vi "OE1311&OE1351_Configure Demodulation.vi"(7 "OE1300_Configure Demodulator":T1={"Demodulator"=1, "Mode"=0, "Arbitrary Frequency"=1000.0, "Harmonic"=1, "Instrument Mode "=4, "Phase  (degree)"=0.0} {"Phase  (degree)" min=-180.0 max=180.0 format="%#.2g"; "Instrument Mode" items=["OE1311"=3, "OE1351"=4, "OE1301"=5]; "Harmonic" min=1 max=32767; "Arbitrary Frequency" min=1e-06 max=1002000.0 format="%#.3f"; "Mode" items=["Harm", "Arb_Freq"]; "Demodulator" items=["1", "2", "3", "4", "5", "6", "7"]}, 8 "Error in (no error)":errorcluster caption="error out（no error）", 9 "Remote Mode":u16(ring)=1 items=["RS232"=1, "Ethernet"=3], 10 "Connection ID in":refnum<k5>, 11 "VISA resource name":refnum<visa-resource-name>) -> (0 "Error out":errorcluster caption="error out", 1 "Output String":string, 2 "Connection ID out":refnum<k5>, 3 "VISA resource  out":refnum<visa-resource-name>)   [LabVIEW 2011]
panel:
  # "Configure \nDemodulator  and Mode"
  # "Configure \nArbitrary Frequency"
  # "Configure Harmonic"
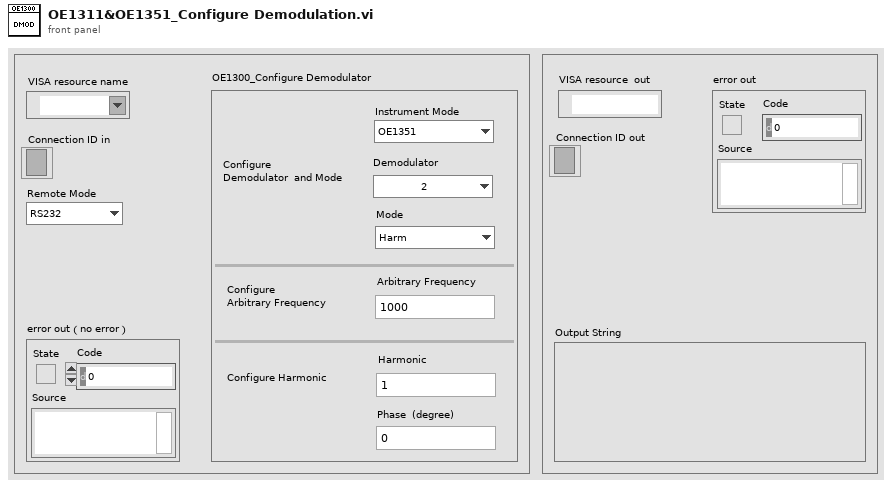
[diagram p1: front panel]
types:
  T1 = cluster{"Demodulator":u16, "Mode":u16, "Arbitrary Frequency":dbl, "Harmonic":u16, "Instrument Mode ":u16, "Phase  (degree)":dbl}
  T2 = enum16{"ISRC", "IGND", "ICPL", "ILIN", "PHAS", "FMOD", "RSLP", "FREQ", "SWPT", "SLLM", "SULM", "SSLL", "SSLG", "STLM", "SWRM", "IRNG", "SENS", "RMOD", "OFLT", "OFSL", "SYNC", "DMOD", "HARM", "DARB", "SWVT", "SLVL", "SVLL", "SVUL", "SVSL", "SVSG", "SVTM", "SVRM", "RALL", "SNAP", "OUTP", "OAUX", "COUT", "CAUX", "COFP", "CEXP", "FPOP", "OEXP", "*IDN", "*RST", "OVLD", "INOV", "GNOV", "*PLL", "SSET", "RSET", "AGAN", "APHS", "ARSV", "ASCL", "EQCD", "EQCS", "SPED", "SRAT", "SLEN", "SSLE", "STRG", "SPRM", "STRD", "PAUS", "REST", "SPTS", "TRCA", "TEMP", "RSTU", "IHNZ", "DEQU", "SADD", "ARNG", "CSPE", "ISRCD", "IGNDD", "ICPLD", "ILIND", "PHASD", "FMODD", "RSLPD", "FREQD", "SWPTD", "SLLMD", "SULMD", "SSLLD", "SSLGD", "STLMD", "SWRMD", "SENSD", "RMODD", "OFLTD", "OFSLD", "SYNCD", "HARMD", "EQCDD", "EQCSD", "SNAPD", "OUTPD", "SWVTD", "SLVLD", "SVLLD", "SVULD", "SVSLD", "SVSGD", "SVTMD", "SVRMD", "SVDCD", "ARSVD", "AGAND", "APHSD", "ASCLD", "FPOPD", "CAUXD", "OEXPD", "SPEDD", "SRATD", "SLEND", "SSLED", "STRGD", "SPRMD", "STRDD", "PAUSD", "RESTD", "SPTSD", "TRCAD", "*IDND", "*RSTD", "INOVD", "GNOVD", "*PLLD", "SSETD", "RSETD", "RALLD"}
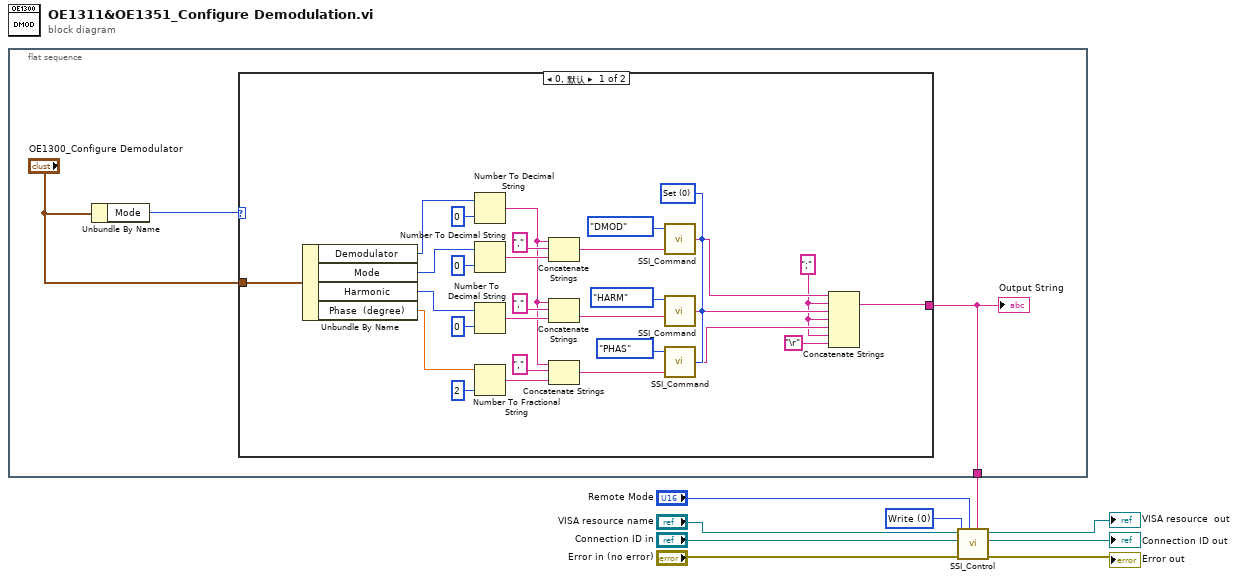
[diagram p0: block diagram]
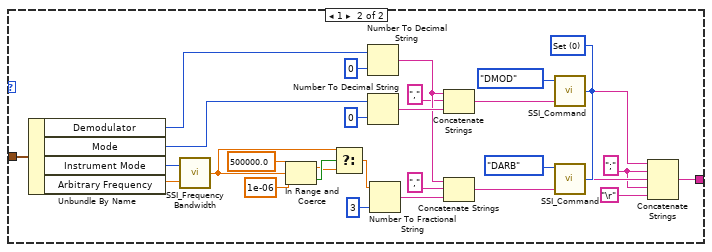
[diagram p2: hidden frame]
diagram:
  w7 = u16 0 items=["Write", "Read"] ("Control")
  n1 = flat-sequence {
    tunnel: [w12] -> w1
    frame #0 {
      n2 = Unbundle By Name("OE1300_Configure Demodulator") -> ("Mode"=w10:u16)
      n3 = case shown="0, 默认" w10 {
        tunnel: [w26 w51] -> w12
        tunnel: "OE1300_Configure Demodulator" -> [w40 w50]
        frame 0, Default {
          w23 = u16 0 items=["Set", "Query"] ("Opera")
          w18 = ";" ("字符串")
          n4 = Unbundle By Name(w40) -> ("Demodulator"=w37:u16, "Mode"=w32:u16, "Harmonic"=w29:u16, "Phase  (degree)"=w20:dbl)
          n5 = Number To Decimal String(number=w37, width (-)=i16 0 ("精度(6)")) -> (decimal integer string=w13:string)
          n6 = Number To Decimal String(number=w32, width (-)=i16 0 ("精度(6)")) -> (decimal integer string=w33:string)
          n7 = Number To Decimal String(number=w29, width (-)=i16 0 ("精度(6)")) -> (decimal integer string=w30:string)
          n8 = Number To Fractional String(number=w20, precision (6)=i16 2 ("精度(6)")) -> (F-format string=w15:string)  [unwired: 2 in]
          n9 = Concatenate Strings(w13, "," ("字符串"), w33) -> (w36:string)
          n10 = Concatenate Strings(w13, "," ("字符串"), w30) -> (w35:string)
          n11 = Concatenate Strings(w13, "," ("字符串"), w15) -> (w14:string)
          n12 = call "SSI_Command.vi"("Opera"=w23, "Paramter"=w36, "Command Type"=T2."DMOD") -> ("Output string"=w28:string)  [unwired: 1 in]
          n13 = call "SSI_Command.vi"("Opera"=w23, "Paramter"=w35, "Command Type"=T2."HARM") -> ("Output string"=w27:string)  [unwired: 1 in]
          n14 = call "SSI_Command.vi"("Opera"=w23, "Paramter"=w14, "Command Type"=T2."PHAS") -> ("Output string"=w19:string)  [unwired: 1 in]
          n15 = Concatenate Strings(w28, w18, w27, w18, w19, w18, "\r") -> (w26:string)
        }
        frame 1 {
          w68 = u16 0 items=["Set", "Query"] ("Opera")
          w56 = ";" ("字符串")
          n16 = Unbundle By Name(w50) -> ("Demodulator"=w66:u16, "Mode"=w61:u16, "Instrument Mode"=w48:u16, "Arbitrary Frequency"=w49:dbl)
          n17 = call "SSI_Frequency Bandwidth.vi"("Frequency"=w49, "Instrument Mode"=w48) -> ("Output"=w43:dbl)  [unwired: 1 in]
          n18 = In Range and Coerce(upper limit=500000.0 ("上限"), x=w43, lower limit=1e-06 ("下限")) -> (coerced(x)=w46:dbl, In Range?=w47:bool)
          n19 = Select(t=w43, s=w47, f=w46) -> (s? t:f=w42:dbl)
          n20 = Number To Decimal String(number=w66, width (-)=i16 0 ("精度(6)")) -> (decimal integer string=w54:string)
          n21 = Number To Decimal String(number=w61, width (-)=i16 0 ("精度(6)")) -> (decimal integer string=w62:string)
          n22 = Number To Fractional String(number=w42, precision (6)=i16 3 ("精度(6)")) -> (F-format string=w59:string)  [unwired: 2 in]
          n23 = Concatenate Strings(w54, "," ("字符串"), w62) -> (w65:string)
          n24 = Concatenate Strings(w54, "," ("字符串"), w59) -> (w64:string)
          n25 = call "SSI_Command.vi"("Opera"=w68, "Paramter"=w65, "Command Type"=T2."DMOD") -> ("Output string"=w58:string)  [unwired: 1 in]
          n26 = call "SSI_Command.vi"("Opera"=w68, "Paramter"=w64, "Command Type"=T2."DARB") -> ("Output string"=w57:string)  [unwired: 1 in]
          n27 = Concatenate Strings(w58, w56, w57, w56, "\r") -> (w51:string)
        }
      }
      "Output String" <- w12
    }
  }
  n28 = call "SSI_Control.vi"("Write Buffer"=w1, "Remote Mode"="Remote Mode", "Error in (no error)"="Error in (no error)", "Control"=w7, "Connection ID in"="Connection ID in", "VISA resource name"="VISA resource name") -> ("Error out"=→"Error out":errorcluster, "Connection ID out"=→"Connection ID out":refnum<k5>, "VISA resource  out"=→"VISA resource  out":refnum<visa-resource-name>)  [unwired: 2 in, 1 out]
